vi "ReadLoop.vi"(11 "notifier":refnum<notifier>) -> ()   [LabVIEW 2022 SP3, in "Acuisition.lvlib"]
uses:
  Acuisition.lvlib
  controls/TaskState.ctl
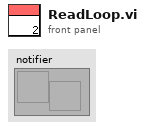
[diagram p1: front panel]
types:
  T1 = typedef "TaskState.ctl" = enum16{"Ready", "Running", "Stopped"}
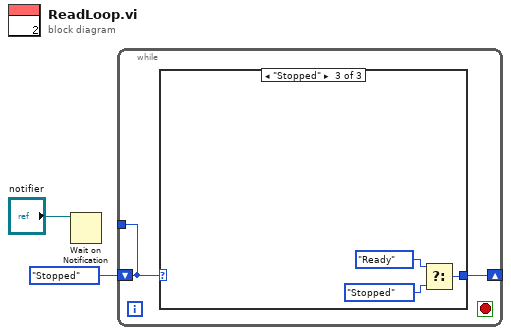
[diagram p0: block diagram]
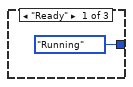
[diagram p2: hidden frame]
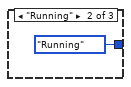
[diagram p3: hidden frame]
diagram:
  n1 = Wait on Notification(notifier="notifier") -> ()  [unwired: 3 in, 4 out]
  n2 = while {
    shift-right: [w4] -> _
    shift-left: TaskState."Stopped" ("States") -> [w3]
    tunnel: [w3] -> _
    stop <- _ stop-if-true
    n3 = case shown="\"Stopped\"" w3 {
      tunnel: [TaskState."Running" ("States") TaskState."Running" ("States") w9] -> w4
      frame "Ready" {
      }
      frame "Running" {
      }
      frame "Stopped" {
        n4 = Select(t=TaskState."Ready" ("States"), f=TaskState."Stopped" ("States")) -> (s? t:f=w9:T1)  [unwired: 1 in]
      }
    }
  }
